vi "SubSystems.vi"(8 "error in":errorcluster) -> ()   [LabVIEW 2016]
doc: "This VI calls the various robot subsystems that will then run in parallel. New subSystems will automatlically script code to make the call."
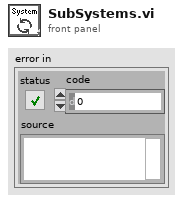
[diagram p1: front panel]
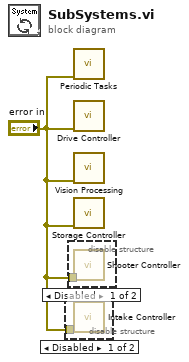
[diagram p0: block diagram]
diagram:
  n1 = disable-structure shown="Disabled" {
    disable-tunnel: "error in" -> [w2 _]
    frame Disabled {
      n2 = call "Intake Controller.vi"("error in"=w2) -> ()  [unwired: 11 in]
    }
    frame Enabled {
    }
  }
  n3 = disable-structure shown="Disabled" {
    disable-tunnel: "error in" -> [w3 _]
    frame Disabled {
      n4 = call "Shooter Controller.vi"("error in"=w3) -> ()  [unwired: 11 in]
    }
    frame Enabled {
    }
  }
  n5 = call "Periodic Tasks.vi"("error in"="error in") -> ()  [unwired: 1 in, 10 out]
  n6 = call "Drive Controller.vi"("error in"="error in") -> ()  [unwired: 11 in]
  n7 = call "Vision Processing.vi"("error in (no error)"="error in") -> ()  [unwired: 7 in]
  n8 = call "Storage Controller.vi"("error in"="error in") -> ()  [unwired: 11 in]
